vi "ramp_simple_1.vi"(5 "array":dbl[](array[numeric]), 6 "treshold":dbl, 7 "time_set":dbl=2.0, 8 "T_sp":dbl=40.0, 9 "master":i32, 10 "reset":i32=1, 11 "pause":i32=1) -> (0 "T control":dbl, 1 "Tr":dbl, 2 "Tin":dbl, 3 "reset_out":dbl, 4 "target_reached":dbl)   [LabVIEW 2017]
uses:
  BERTTA.dll
panel:
  out "element":i32
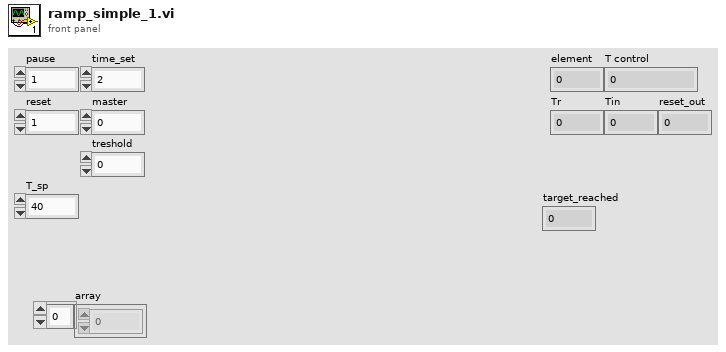
[diagram p1: front panel]
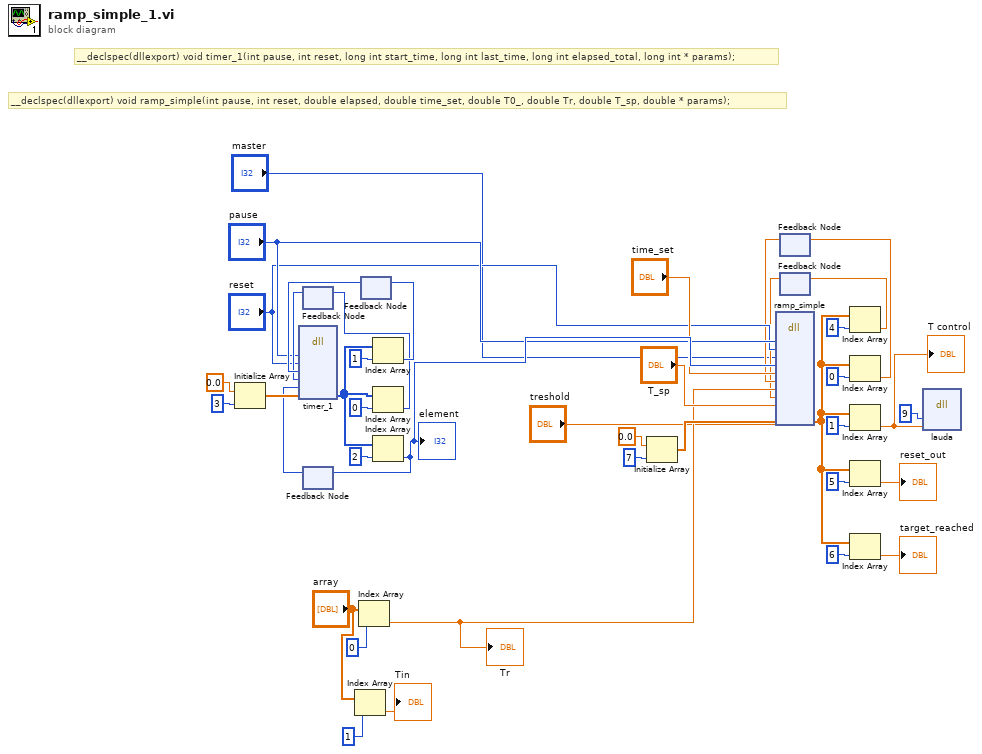
[diagram p0: block diagram]
diagram:
  # "__declspec(dllexport) void ramp_simple(int pause, int reset, double elapsed, double time_set, double T0_, double Tr, double T_sp, double * params);"
  # "__declspec(dllexport) void timer_1(int pause, int reset, long int start_time, long int last_time, long int elapsed_total, long int * params);"
  n1 = Initialize Array(0.0 ("element"), 3 ("dimension size")) -> (w41:dbl[])
  n2 = feedback #1() -> (w30:i32)  [unwired: 1 in]
  n3 = feedback #2() -> (w34:i32)  [unwired: 1 in]
  n4 = Index Array(array="array", index=1) -> (element=→"Tin":dbl)
  n5 = Index Array(array="array", index=0) -> (element=w16:dbl)
  "Tr" <- w16
  n6 = feedback #3() -> (w32:i32)  [unwired: 1 in]
  n7 = dll-call lib="C:/Users/shresplab/OneDrive - Kemira Oyj/Documents/GitHub/Bertta/BERTTA/x64/Debug/BERTTA.dll" fn="timer_1"("pause"="pause", "reset"="reset", "start_time"=w32, "last_time"=w30, "elapsed_total"=w34, "params"=w41) -> ("params"=w35:i32[])  [unwired: 9 in, 2 out]
  n8 = Index Array(array=w35, index=1) -> (element=w33:i32)
  n9 = feedback-in #3(w33) -> ()
  n10 = Index Array(array=w35, index=0) -> (element=w31:i32)
  n11 = feedback-in #1(w31) -> ()
  n12 = Index Array(array=w35, index=2) -> (element=w29:i32)
  "element" <- w29
  n13 = feedback-in #2(w29) -> ()
  n14 = Initialize Array(0.0 ("element"), 7 ("dimension size")) -> (w26:dbl[])
  n15 = feedback #4() -> (w18:dbl)  [unwired: 1 in]
  n16 = feedback #5() -> (w8:dbl)  [unwired: 1 in]
  n17 = dll-call lib="C:/Users/shresplab/OneDrive - Kemira Oyj/Documents/GitHub/Bertta/BERTTA/x64/Debug/BERTTA.dll" fn="ramp_simple"("pause"="pause", "reset"="reset", "master"="master", "elapsed"=w29, "time_set"="time_set", "T0_"=w18, "Tr"=w16, "Tr_last"=w8, "T_sp"="T_sp", "treshold"="treshold", "params"=w26) -> ("params"=w1:dbl[])  [unwired: 14 in, 2 out]
  n18 = Index Array(array=w1, index=4) -> (element=w9:dbl)
  n19 = feedback-in #5(w9) -> ()
  n20 = Index Array(array=w1, index=0) -> (element=w19:dbl)
  n21 = feedback-in #4(w19) -> ()
  n22 = Index Array(array=w1, index=1) -> (element=w11:dbl)
  "T control" <- w11
  n23 = Index Array(array=w1, index=5) -> (element=→"reset_out":dbl)
  n24 = Index Array(array=w1, index=6) -> (element=→"target_reached":dbl)
  n25 = dll-call lib="C:/Users/shresplab/OneDrive - Kemira Oyj/Documents/GitHub/Bertta/BERTTA/x64/Debug/BERTTA.dll" fn="lauda"("port"=9, "set_temp"=w11) -> ()  [unwired: 6 in, 2 out]
